vi "Show Message Log MHLC.vi"(8 "error in (no error)":errorcluster, 10 "Data in":variant, 11 "Debug Server in":refnum<class "Debug Server.lvclass">) -> (0 "error out":errorcluster, 3 "Debug Server out":refnum<class "Debug Server.lvclass">)   [LabVIEW 2017, in "Debug Server.lvclass"]
doc: "If the requested Message Log already exists, open its front panel.\nOtherwise, load a new Message Log for the selected Worker."
uses:
  Debug Server.lvclass
  C:/Program Files (x86)/National Instruments/LabVIEW 2017/vi.lib/addons/_Workers/Library/Classes/Worker/Worker.lvclass
  Debug Server.lvclass/Debug Server.ctl
  Dynamic Message Log Data.ctl
  Message Log/Message Log.lvclass
  Common VIs/DC_UID.ctl
  Common VIs/Message Log ID.ctl
  Debug Server TCP Server and Client/Workers/DS TCP Server/rqp_Message Log Ready.ctl
  <vilib>/addons/_Workers/Library/Classes/Message Queue/Message Queue.lvclass
  Message Log/Initialization Data.ctl
  Message Log/Response Cases.ctl
  <vilib>/addons/_Workers/Library/Case Label.ctl
  Message Log/Config Data.ctl
  <vilib>/Utility/miscctls.llb/LVRectTypeDef.ctl
  <vilib>/addons/_Workers/Library/Classes/Worker/Worker.lvclass/Worker.ctl
  Application Manager/Application Manager.lvclass
  Debug Server TCP Server and Client/Workers/DS TCP Server/DS TCP Server.lvclass
  <vilib>/addons/_Workers/Library/Classes/Worker/Worker.lvclass
  <vilib>/addons/_Workers/Library/Workers.lvlib
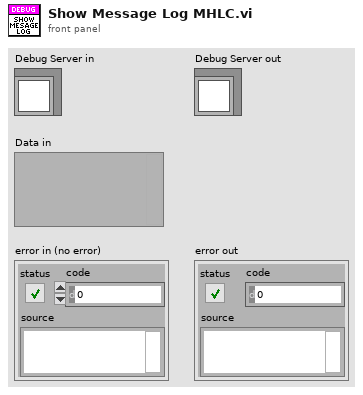
[diagram p1: front panel]
types:
  T1 = typedef "Application Manager.lvclass/rsp_Show Message Log.ctl" = cluster{"DC_UID":T2, "Head Worker ID":string, "IP Address":string}
  T2 = typedef "DC_UID.ctl" = string
  T3 = typedef "Debug Server.lvclass/Dynamic Message Log Data.ctl" = cluster{"Message Log":refnum<class "Message Log.lvclass">, "DC_UID":T2, "Message Log ID":T4}
  T4 = typedef "Message Log ID.ctl" = cluster{"Head Worker ID":string, "IP Address":string}
  T5 = typedef "Message Log.lvclass/Initialization Data.ctl" = cluster{"Response Cases":T6, "Message Log ID":T4, "Config Data":T8}
  T6 = typedef "Message Log.lvclass/Response Cases.ctl" = cluster{"Message Log Exited":T7, "Go to MHL Case":T7, "Open Running VI":T7, "Message Log Shutdown Data":T7, "Show Application Manager":T7}
  T7 = typedef "Workers.lvlib/Case Label.ctl" = string
  T8 = typedef "Message Log.lvclass/Config Data.ctl" = cluster{"Max Num Rows":i32, "Visible Columns":bool[], "Splitter Position":i32, "Column Widths":u32[], "WinBounds":T9, "FP.State":enum32{"Invalid", "Standard", "Closed", "Hidden", "Minimized", "Maximized"}, "Monitor":u16, "Logging":bool, "LogBaseFolder":path}
  T9 = typedef "LVRectTypeDef.ctl" = cluster{"Left":i16, "Top":i16, "Right":i16, "Bottom":i16}
  T10 = typedef "DS TCP Server.lvlib/DS TCP Server.lvclass/rqp_Message Log Ready.ctl" = cluster{"Message Log Q":refnum<class "Message Queue.lvclass">, "Message Log ID":T4, "DC_UID":T2}
  T11 = enum32{"Invalid", "Standard", "Closed", "Hidden", "Minimized", "Maximized"}
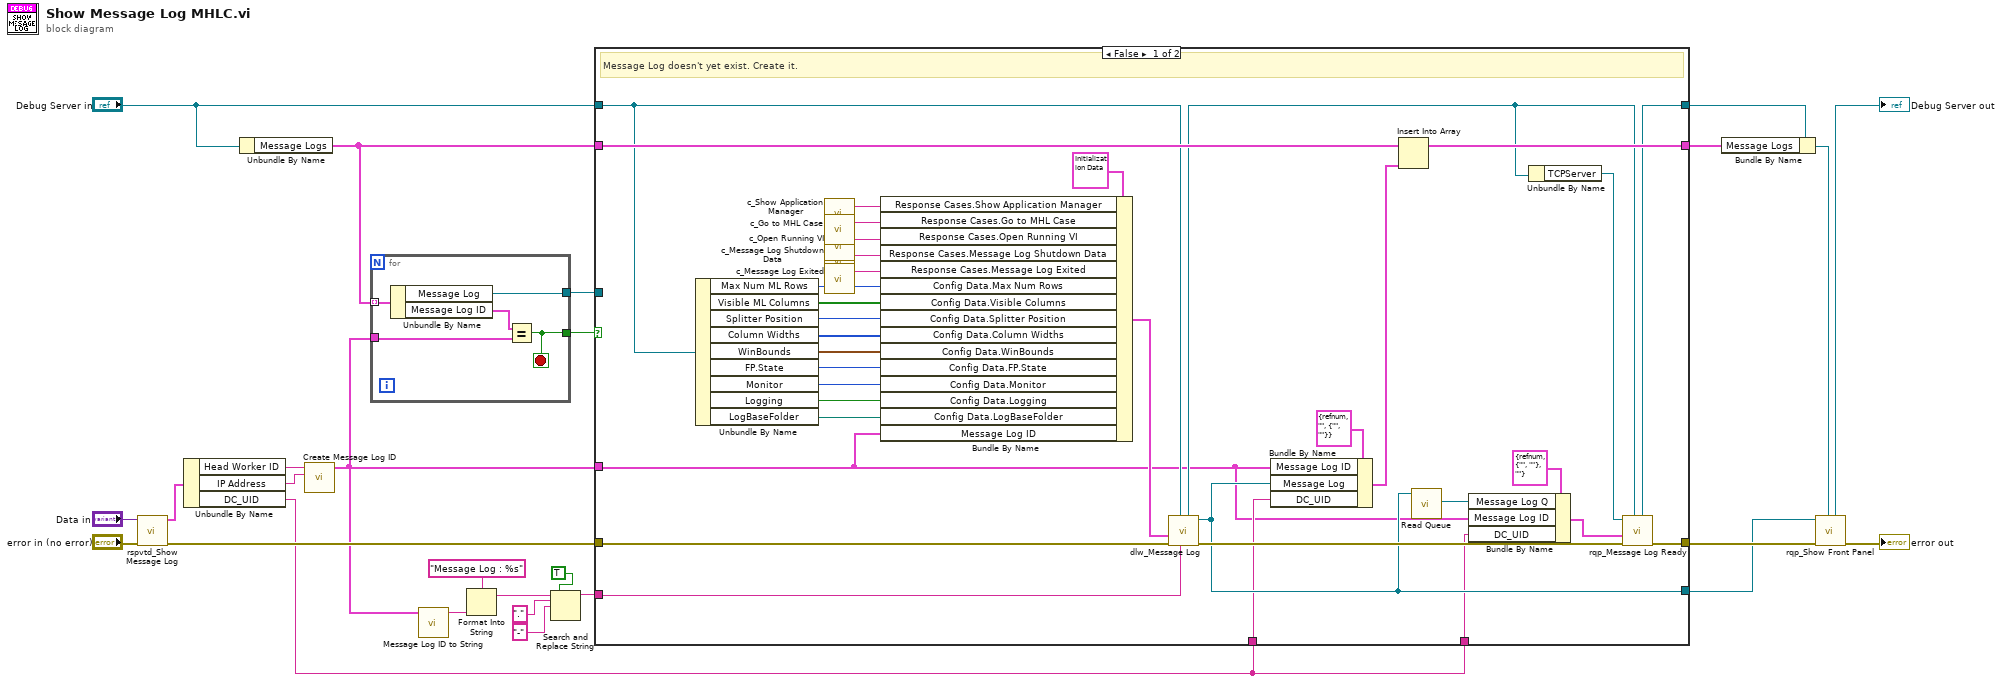
[diagram p0: block diagram]
diagram:
  n1 = call "rspvtd_Show Message Log.vi"("error in"="error in (no error)", "Data in"="Data in") -> ("error out"=w22:errorcluster, "Data out"=w26:T1)  [unwired: 8 in]
  n2 = Unbundle By Name(w26) -> ("Head Worker ID"=w4:string, "IP Address"=w3:string, "DC_UID"=w5:T2)
  n3 = Unbundle By Name("Debug Server in") -> ("Message Logs"=w18:T3[])
  n4 = call "Create Message Log ID.vi"("IP Address"=w3, "Head Worker WID"=w4) -> ("Message Log ID"=w1:T4)  [unwired: 9 in]
  n5 = for {
    tunnel: w18 -> [w31] mode=indexing
    tunnel: w1 -> [w29]
    tunnel: [w28] -> w20
    tunnel: [w27] -> w14
    stop <- w28 stop-if-true
    n6 = Unbundle By Name(w31) -> ("Message Log"=w27:refnum<class "Message Log.lvclass">, "Message Log ID"=w30:T4)
    n7 = Equal?(x=w30, y=w29) -> (x = y?=w28:bool)
  }
  n8 = call "Message Log ID to String.vi"("Message Log ID"=w1) -> ("Message Log ID String"=w2:string)  [unwired: 10 in]
  n9 = Format Into String(format string="Message Log : %s", w2) -> (resulting string=w9:string)  [unwired: 2 in, 1 out]
  n10 = Search and Replace String(replace all?=TRUE ("replace all? (F)"), input string=w9, search string=".", replace string="-" ("replace string (\"\")")) -> (result string=w8:string)  [unwired: 4 in, 3 out]
  n11 = case shown="False" w20 {
    tunnel: "Debug Server in" -> [w49 w69]
    tunnel: [w54 w69] -> w17
    tunnel: w22 -> [w66 w70]
    tunnel: [w57 w70] -> w21
    tunnel: w8 -> [w64 _]
    tunnel: w18 -> [w63 w68]
    tunnel: [w62 w68] -> w16
    tunnel: w1 -> [w46 _]
    tunnel: [w59 w67] -> w13
    tunnel: w14 -> [_ w67]
    tunnel: w5 -> [w51 _]
    tunnel: w5 -> [w50 _]
    frame False {
      # "Message Log doesn't yet exist. Create it."
      n12 = Unbundle By Name(w49) -> ("Max Num ML Rows"=w44:i32, "Visible ML Columns"=w43:bool[], "Splitter Position"=w42:i32, "Column Widths"=w41:u32[], "WinBounds"=w40:T9, "FP.State"=w39:T11, "Monitor"=w38:u16, "Logging"=w33:bool, "LogBaseFolder"=w32:path)
      n13 = call "c_Show Application Manager.vi"() -> ("Case Label"=w34:T7)  [unwired: 1 in]
      n14 = call "c_Go to MHL Case.vi"() -> ("Case Label"=w36:T7)  [unwired: 1 in]
      n15 = call "c_Open Running VI.vi"() -> ("Case Label"=w37:T7)  [unwired: 1 in]
      n16 = call "c_Message Log Shutdown Data.vi"() -> ("Case Label"=w35:T7)  [unwired: 1 in]
      n17 = call "c_Message Log Exited.vi"() -> ("Case Label"=w45:T7)  [unwired: 1 in]
      n18 = Bundle By Name(cluster=T5 {"Response Cases"={"Message Log Exited"="", "Go to MHL Case"="", "Open Running VI"="", "Message Log Shutdown Data"="", "Show Application Manager"=""}, "Message Log ID"={"Head Worker ID"="", "IP Address"=""}, "Config Data"={"Max Num Rows"=0, "Visible Columns"=[], "Splitter Position"=0, "Column Widths"=[], "WinBounds"={"Left"=0, "Top"=0, "Right"=0, "Bottom"=0}, "FP.State"=enum."Invalid", "Monitor"=0, "Logging"=FALSE, "LogBaseFolder"=path ""}} ("Initialization Data"), "Response Cases.Show Application Manager"=w34, "Response Cases.Go to MHL Case"=w36, "Response Cases.Open Running VI"=w37, "Response Cases.Message Log Shutdown Data"=w35, "Response Cases.Message Log Exited"=w45, "Config Data.Max Num Rows"=w44, "Config Data.Visible Columns"=w43, "Config Data.Splitter Position"=w42, "Config Data.Column Widths"=w41, "Config Data.WinBounds"=w40, "Config Data.FP.State"=w39, "Config Data.Monitor"=w38, "Config Data.Logging"=w33, "Config Data.LogBaseFolder"=w32, "Message Log ID"=w46) -> (w48:T5)
      n19 = call "dlw_Message Log.vi"("Worker Alias"=w64, "Caller in"=w49, "error in"=w66, "Initialization Data"=w48) -> ("error out"=w65:errorcluster, "Message Log out"=w59:refnum<class "Message Log.lvclass">, "dup Caller out"=w53:refnum<class "Debug Server.lvclass">)  [unwired: 5 in]
      n20 = Bundle By Name(cluster=T3 {"Message Log"=refnum, "DC_UID"="", "Message Log ID"={"Head Worker ID"="", "IP Address"=""}} ("Data"), "Message Log ID"=w46, "Message Log"=w59, "DC_UID"=w50) -> (w60:T3)
      n21 = Insert Into Array(array=w63, new element=w60) -> (w62:T3[])  [unwired: 1 in]
      n22 = call <vilib>:"Read Queue.vi"("Worker_"=w59) -> ("Message Queue out"=w58:refnum<class "Message Queue.lvclass">)  [unwired: 9 in, 1 out]
      n23 = Bundle By Name(cluster=T10 {"Message Log Q"=refnum, "Message Log ID"={"Head Worker ID"="", "IP Address"=""}, "DC_UID"=""} ("Data in"), "Message Log Q"=w58, "Message Log ID"=w46, "DC_UID"=w51) -> (w55:T10)
      n24 = Unbundle By Name(w53) -> ("TCPServer"=w52:refnum<class "DS TCP Server.lvclass">)
      n25 = call "rqp_Message Log Ready.vi"("Caller in"=w53, "error in"=w65, "Data in"=w55, "DS TCP Server in"=w52) -> ("error out"=w57:errorcluster, "dup Caller out"=w54:refnum<class "Debug Server.lvclass">)  [unwired: 5 in, 1 out]
    }
    frame True {
      # "Message Log already exists. Do nothing."
    }
  }
  n26 = Bundle By Name(cluster=w17, "Message Logs"=w16) -> (w15:refnum<class "Debug Server.lvclass">)
  n27 = call "rqp_Show Front Panel.vi"("Caller in"=w15, "error in"=w21, "Message Log in"=w13) -> ("error out"=→"error out":errorcluster, "dup Caller out"=→"Debug Server out":refnum<class "Debug Server.lvclass">)  [unwired: 6 in, 1 out]
